vi "Code String LV Example.vi"() -> ()   [LabVIEW 2016]
doc: "LabVIEW Code String example.\n--------------------\nCopyright (c) 2019 Analog Devices, Inc. All rights reserved.\n\nRedistribution and use in source and binary forms, with or without modification,\nare permitted provided that the following conditions are met:\n - Redistributions of source code must retain the above copyright notice, this\n list of conditions and the following disclaimer.\n - Redistributions in binary form must reproduce the above copyright notice,\n this list of conditions and the following disclaimer in the documentation\n and/or other materials provided with the distribution.\n - Modified versions of the software must be conspicuously marked as such.\n - This software is licensed solely and exclusively for use with\n processors/products manufactured by or for Analog Devices, Inc.\n - This software may not be combined or merged with other code in any manner\n that would cause the software to become subject to terms and conditions\n which differ from those listed here.\n - Neither the name of Analog Devices, Inc. nor the names of its contributors\n may be used to endorse or promote products derived from this software\n without specific prior written permission.\n - The use of this software may or may not infringe the patent rights of one or\n more patent holders. This license does not release you from the requirement\n that you obtain separate licenses from these patent holders to use this\n software.\n\nTHIS SOFTWARE IS PROVIDED BY ANALOG DEVICES, INC. AND CONTRIBUTORS \"AS IS\" AND\nANY EXPRESS OR IMPLIED WARRANTIES, INCLUDING, BUT NOT LIMITED TO,\nNON-INFRINGEMENT, TITLE, MERCHANTABILITY AND FITNESS FOR A PARTICULAR PURPOSE\nARE DISCLAIMED. IN NO EVENT SHALL ANALOG DEVICES, INC. OR CONTRIBUTORS BE LIABLE\nFOR ANY DIRECT, INDIRECT, INCIDENTAL, SPECIAL, EXEMPLARY, PUNITIVE OR\nCONSEQUENTIAL DAMAGES (INCLUDING, BUT NOT LIMITED TO, DAMAGES ARISING OUT OF\nCLAIMS OF INTELLECTUAL PROPERTY RIGHTS INFRINGEMENT; PROCUREMENT OF SUBSTITUTE\nGOODS OR SERVICES; LOSS OF USE, DATA, OR PROFITS; OR BUSINESS INTERRUPTION)\nHOWEVER CAUSED AND ON ANY THEORY OF LIABILITY, WHETHER IN CONTRACT, STRICT\nLIABILITY, OR TORT (INCLUDING NEGLIGENCE OR OTHERWISE) ARISING IN ANY WAY OUT OF\nTHE USE OF THIS SOFTWARE, EVEN IF ADVISED OF THE POSSIBILITY OF SUCH DAMAGE.\n\n2019-01-10-7CBSD SLA"
uses:
  library/Code String/Code String/Code String.lvclass/Code String.ctl
  library/Code String/Code String LV/Code String LV.lvclass
  C:/Git/ipn_lv_dev/code-string/source/library/Code String/Code String/Code String.lvclass
  library/Code String/Code String LV/Create Code String LV.vi
  library/Code String/Code String/Properties/Write Keywords.vi
  library/Code String/Code String/Properties/Write Font Size.vi
  library/Code String/Code String/Properties/Write Completion.vi
  library/Code String/Code String/Properties/Write Delimiter Pattern.vi
  library/Code String/Code String/Properties/Write Editable.vi
  library/Code String/Code String/Properties/Write Selected Text.vi
  library/Code String/Code String/Properties/Write Font Color.vi
  library/Code String/Code String/Properties/Write Selection End.vi
  library/Code String/Code String/Properties/Write Selection Start.vi
  library/Code String/Code String/Properties/Read Selected Line(s).vi
  library/Code String/Code String/Properties/Read Selected Token.vi
  library/Code String/Code String/Properties/Read # Selected Lines.vi
  library/Code String/Code String/Properties/Read Selected Text.vi
  library/Code String/Code String/Code String.lvclass
panel:
  in  "Replacement Text":string="Test"
  in  "Replace Selection":bool
  out "Selected Text":string
  out "# Lines":i32
  out "Selected Token":string
  out "Selected Line(s)":string
  in  "Auto-complete":bool=TRUE
  in  "Editable":bool=TRUE
  in  "Checked?":bool
  out "Selected Menu Item":string
  in  "Item Name/Tag":string
  in  "Visible?":bool
  in  "Set Menu Item":bool
  in  "Selection End":u32
  in  "Selection Start":u32
  in  "Font Color":u32(colorbox)
  in  "Font Size":u32=14
  # "Copyright (c) 2019 Analog Devices, Inc.  All rights reserved.\n\nRedistribution and use in source and binary forms, with or without modification,\nare permitted provided that the following conditions are met:\n  - Redistributions of source code must retain the above copyright notice, this\n    list of conditions and the following disclaimer.\n  - Redistributions in binary form must reproduce the above copyright notice,\n    this list of conditions and the following disclaimer in the documentation\n    and/or other materials provided with the distribution.\n  - Modified versions of the software must be conspicuously marked as such.\n  - This software is licensed solely and exclusively for use with\n    processors/products manufactured by or for Analog Devices, Inc.\n  - This software may not be combined or merged with other code in any manner\n    that would cause the software to become subject to terms and conditions\n    which differ from those listed here.\n  - Neither the name of Analog Devices, Inc. nor the names of its contributors\n    may be used to endorse or promote products derived from this software\n    without specific prior written permission.\n  - The use of this software may or may not infringe the patent rights of one or\n    more patent holders.  This license does not release you from the requirement\n    that you obtain separate licenses from these patent holders to use this\n    software.\n\nTHIS SOFTWARE IS PROVIDED BY ANALOG DEVICES, INC. AND CONTRIBUTORS \"AS IS\" AND\nANY EXPRESS OR IMPLIED WARRANTIES, INCLUDING, BUT NOT LIMITED TO,\nNON-INFRINGEMENT, TITLE, MERCHANTABILITY AND FITNESS FOR A PARTICULAR PURPOSE\nARE DISCLAIMED. IN NO EVENT SHALL ANALOG DEVICES, INC. OR CONTRIBUTORS BE LIABLE\nFOR ANY DIRECT, INDIRECT, INCIDENTAL, SPECIAL, EXEMPLARY, PUNITIVE OR\nCONSEQUENTIAL DAMAGES (INCLUDING, BUT NOT LIMITED TO, DAMAGES ARISING OUT OF\nCLAIMS OF INTELLECTUAL PROPERTY RIGHTS INFRINGEMENT; PROCUREMENT OF SUBSTITUTE\nGOODS OR SERVICES; LOSS OF USE, DATA, OR PROFITS; OR BUSINESS INTERRUPTION)\nHOWEVER CAUSED AND ON ANY THEORY OF LIABILITY, WHETHER IN CONTRACT, STRICT\nLIABILITY, OR TORT (INCLUDING NEGLIGENCE OR OTHERWISE) ARISING IN ANY WAY OUT OF\nTHE USE OF THIS SOFTWARE, EVEN IF ADVISED OF THE POSSIBILITY OF SUCH DAMAGE.\n\n2019-01-10-7CBSD SLA"
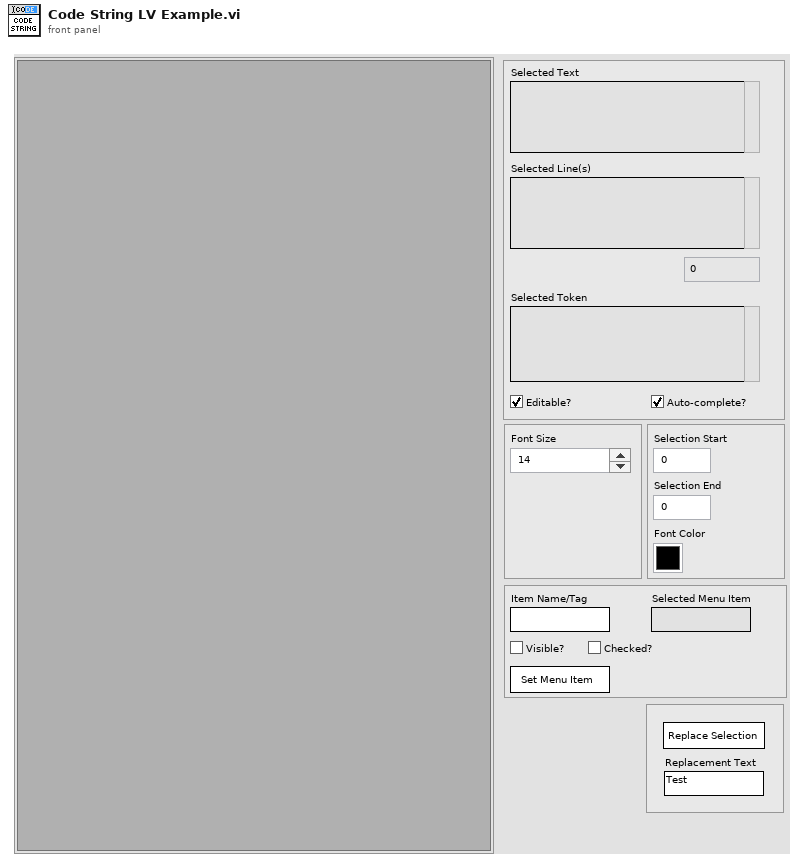
[diagram p1: front panel]
types:
  T1 = typedef "Code String.lvclass/Public Events.ctl" = cluster{"Selected Token Changed":refnum<user-event>, "Value Changed":refnum<user-event>, "Shortcut Menu Selection":refnum<user-event>}
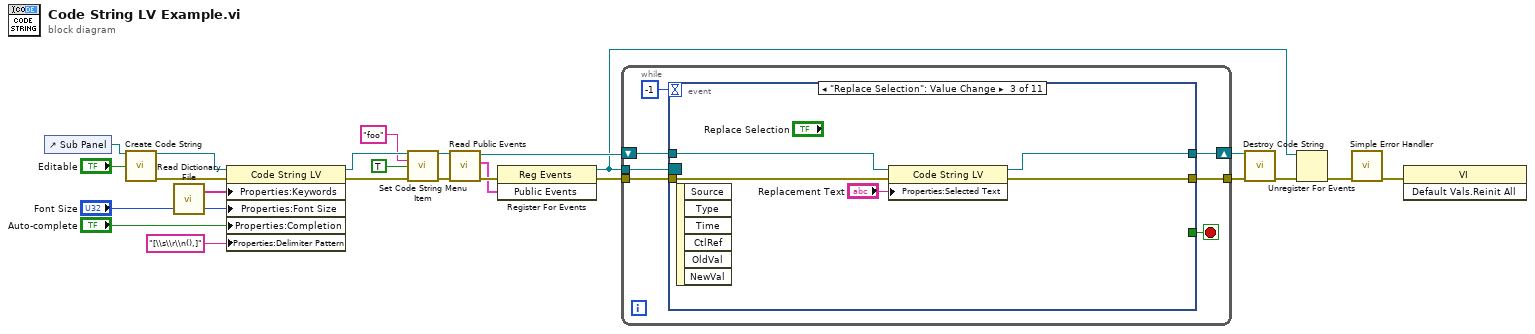
[diagram p0: block diagram]
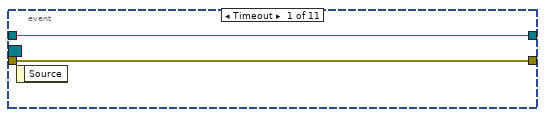
[diagram p2: hidden frame]
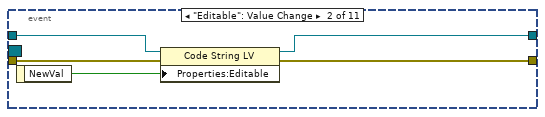
[diagram p3: hidden frame]
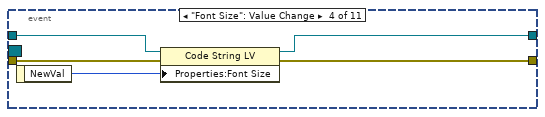
[diagram p4: hidden frame]
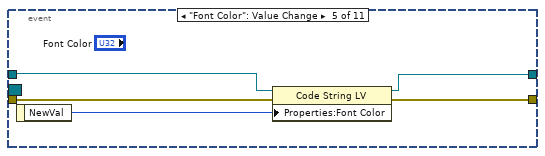
[diagram p5: hidden frame]
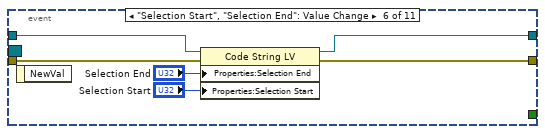
[diagram p6: hidden frame]
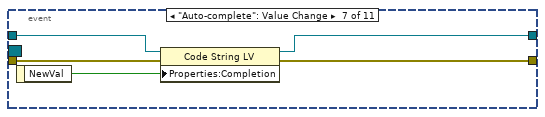
[diagram p7: hidden frame]
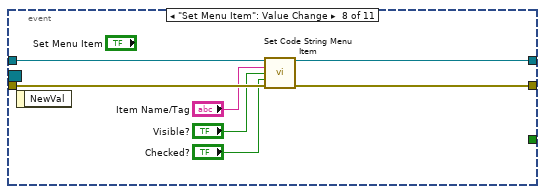
[diagram p8: hidden frame]
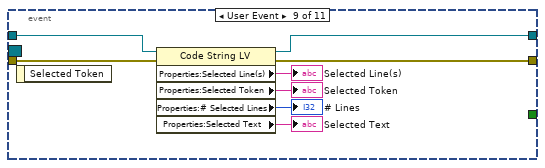
[diagram p9: hidden frame]
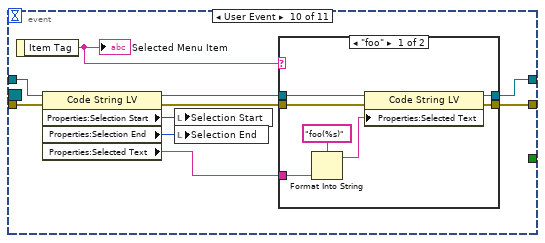
[diagram p10: hidden frame]
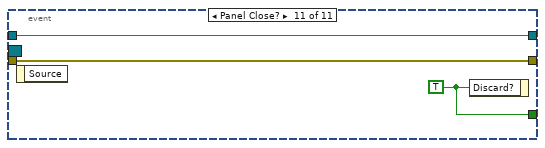
[diagram p12: hidden frame]
diagram:
  n1 = control-ref of="Sub Panel"() -> (w7:refnum<vi>)
  n2 = call-poly "Create Code String.vi"("Subpanel"=w7, "Editable? (T)"="Editable") -> ("Code String LV"=w24:refnum<class "Code String LV.lvclass">, "error out"=w20:errorcluster)  [unwired: 12 in]
  n3 = call "Read Dictionary File.vi"() -> ("dictionary"=w9:string[])  [unwired: 3 in]
  n4 = property class="Code String LV"(reference=w24, error in=w20, "Properties:Keywords"=w9, "Properties:Font Size"="Font Size", "Properties:Completion"="Auto-complete", "Properties:Delimiter Pattern"="[\\s\\r\\n(),]") -> (reference out=w4:refnum<class "Code String LV.lvclass">, error out=w19:errorcluster)
  n5 = call "Set Code String Menu Item.vi"("Code String in"=w4, "Item Path"="foo", "Visibility (T)"=TRUE, "error in (no error)"=w19) -> ("Code String out"=w3:refnum<class "Code String LV.lvclass">, "error out"=w5:errorcluster)  [unwired: 10 in]
  n6 = call "Read Public Events.vi"("error in (no error)"=w5, "Code String in"=w3) -> ("error out"=w16:errorcluster, "Public Events"=w13:T1, "Code String out"=w15:refnum<class "Code String LV.lvclass">)  [unwired: 7 in]
  n7 = register-events(error in=w16, w13) -> (reference out=w10:refnum<event-registration>, error out=w14:errorcluster)  [unwired: 1 in]
  n8 = while {
    shift-right: [w30] -> w23
    shift-left: w15 -> [w31]
    tunnel: w14 -> [w29]
    tunnel: [w28] -> w22
    tunnel: w10 -> [w25]
    stop <- w26 stop-if-true
    n9 = event shown="[2] \"Replace Selection\": Value Change" {
      selector: w25 -> [_ _ _ _ _ _ _ _ _ _ _]
      dyn-events: _ -> [_ _ _ _ _ _ _ _ _ _ _]
      timeout: -1 -> [_ _ _ _ _ _ _ _ _ _ _]
      tunnel: w31 -> [w33 w37 w41 w46 w49 w57 w62 w69 w77 w88 w99]
      tunnel: [w33 w36 w40 w45 w51 w56 w61 w68 w76 w81 w99] -> w30
      tunnel: w29 -> [w32 w38 w43 w48 w53 w59 w64 w71 w75 w89 w100]
      tunnel: [w32 w35 w42 w47 w52 w58 w63 w70 w74 w80 w100] -> w28
      tunnel: [_ _ _ _ _ _ _ _ _ _ w101] -> w26
      event Timeout {
        n10 = event-data() -> ()  [unwired: 1 in, 1 out]
      }
      event "Editable": Value Change {
        n11 = event-data() -> ("NewVal"=w34:bool)  [unwired: 1 in]
        n12 = property class="Code String LV"(reference=w37, error in=w38, "Properties:Editable"=w34) -> (reference out=w36:refnum<class "Code String LV.lvclass">, error out=w35:errorcluster)
      }
      event "Replace Selection": Value Change {
        n13 = event-data() -> ()  [unwired: 1 in, 6 out]
        n14 = property class="Code String LV"(reference=w41, error in=w43, "Properties:Selected Text"="Replacement Text") -> (reference out=w40:refnum<class "Code String LV.lvclass">, error out=w42:errorcluster)
      }
      event "Font Size": Value Change {
        n15 = event-data() -> ("NewVal"=w44:u32)  [unwired: 1 in]
        n16 = property class="Code String LV"(reference=w46, error in=w48, "Properties:Font Size"=w44) -> (reference out=w45:refnum<class "Code String LV.lvclass">, error out=w47:errorcluster)
      }
      event "Font Color": Value Change {
        n17 = event-data() -> ("NewVal"=w50:u32)  [unwired: 1 in]
        n18 = property class="Code String LV"(reference=w49, error in=w53, "Properties:Font Color"=w50) -> (reference out=w51:refnum<class "Code String LV.lvclass">, error out=w52:errorcluster)
      }
      event "Selection Start", "Selection End": Value Change {
        n19 = event-data() -> ()  [unwired: 1 in, 1 out]
        n20 = property class="Code String LV"(reference=w57, error in=w59, "Properties:Selection End"="Selection End", "Properties:Selection Start"="Selection Start") -> (reference out=w56:refnum<class "Code String LV.lvclass">, error out=w58:errorcluster)
      }
      event "Auto-complete": Value Change {
        n21 = event-data() -> ("NewVal"=w60:bool)  [unwired: 1 in]
        n22 = property class="Code String LV"(reference=w62, error in=w64, "Properties:Completion"=w60) -> (reference out=w61:refnum<class "Code String LV.lvclass">, error out=w63:errorcluster)
      }
      event "Set Menu Item": Value Change {
        n23 = event-data() -> ()  [unwired: 1 in, 1 out]
        n24 = call "Set Code String Menu Item.vi"("Code String in"=w69, "Item Path"="Item Name/Tag", "Visibility (T)"="Visible?", "Checked (F)"="Checked?", "error in (no error)"=w71) -> ("Code String out"=w68:refnum<class "Code String LV.lvclass">, "error out"=w70:errorcluster)  [unwired: 9 in]
      }
      event User Event {
        n25 = event-data() -> ()  [unwired: 1 in, 1 out]
        n26 = property class="Code String LV"(reference=w77, error in=w75) -> (reference out=w76:refnum<class "Code String LV.lvclass">, error out=w74:errorcluster, "Properties:Selected Line(s)"=→"Selected Line(s)":string, "Properties:Selected Token"=→"Selected Token":string, "Properties:# Selected Lines"=→"# Lines":i32, "Properties:Selected Text"=→"Selected Text":string)
      }
      event User Event {
        n27 = event-data() -> ("Item Tag"=w85:string)  [unwired: 1 in]
        "Selected Menu Item" <- w85
        n28 = property class="Code String LV"(reference=w88, error in=w89) -> (reference out=w82:refnum<class "Code String LV.lvclass">, error out=w83:errorcluster, "Properties:Selection Start"=w86:u32, "Properties:Selection End"=w87:u32, "Properties:Selected Text"=w84:string)
        n29 = local write "Selection Start"(w86) -> ()
        n30 = local write "Selection End"(w87) -> ()
        n31 = case shown="\"foo\"" w85 {
          tunnel: w84 -> [w96 _]
          tunnel: w83 -> [w94 w98]
          tunnel: w82 -> [w93 w97]
          tunnel: [w92 w97] -> w81
          tunnel: [w90 w98] -> w80
          frame "foo" {
            n32 = Format Into String(format string="foo(%s)", w96) -> (resulting string=w91:string)  [unwired: 2 in, 1 out]
            n33 = property class="Code String LV"(reference=w93, error in=w94, "Properties:Selected Text"=w91) -> (reference out=w92:refnum<class "Code String LV.lvclass">, error out=w90:errorcluster)
          }
          frame Default {
          }
        }
      }
      event Panel Close? {
        w101 = TRUE ("Discard?")
        n34 = event-data() -> ()  [unwired: 1 in, 1 out]
        n35 = event-data("Discard?"=w101) -> ()  [unwired: 1 in, 1 out]
      }
    }
  }
  n36 = call "Destroy Code String.vi"("Code String in"=w23, "error in (no error)"=w22) -> ("error out"=w21:errorcluster)  [unwired: 12 in, 1 out]
  n37 = Unregister For Events(event registration refnum=w10, error in=w21) -> (error out=w11:errorcluster)
  n38 = call <vilib>:"Simple Error Handler.vi"("error in (no error)"=w11) -> ("error out"=w6:errorcluster)  [unwired: 4 in, 4 out]
  n39 = invoke class="VI" method="Default Vals.Reinit All"(error in=w6) -> ()  [unwired: 2 in, 3 out]
